vi "Init.vi"(8 "error in (no error)":errorcluster, 11 "LHL Actor in":refnum<class "LHL Actor.lvclass">) -> (0 "error out":errorcluster, 3 "LHL Actor out":refnum<class "LHL Actor.lvclass">)   [LabVIEW 2020, in "LHL Actor.lvlib" / "LHL Actor.lvclass"]
uses:
  LHL Actor.lvclass
  LHL Actor.lvclass/LHL Actor.ctl
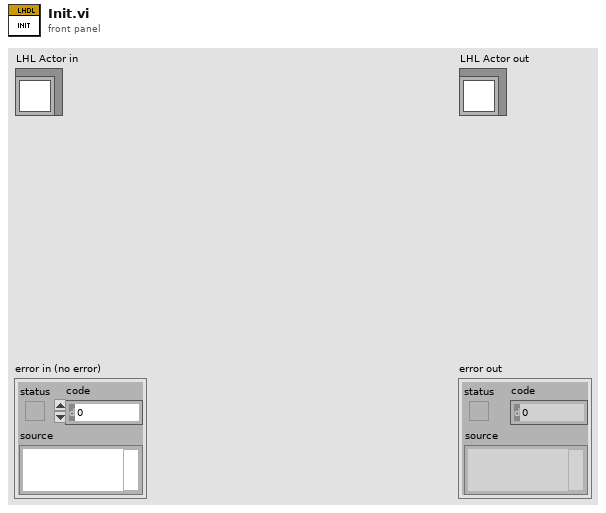
[diagram p1: front panel]
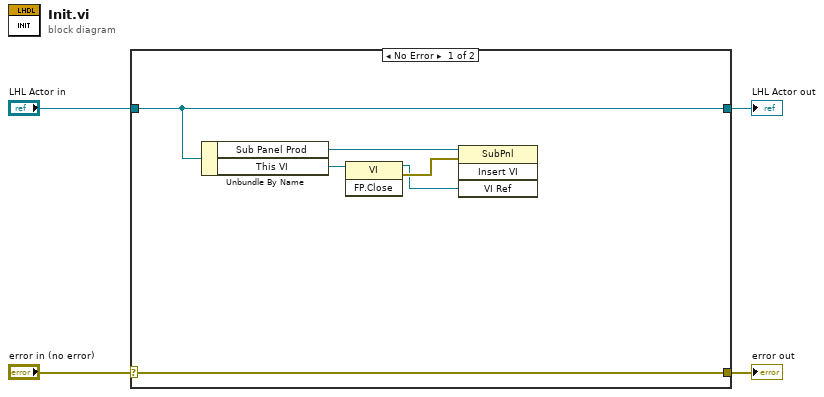
[diagram p0: block diagram]
diagram:
  n1 = case shown="No Error" "error in (no error)" {
    selector: "error in (no error)" -> [w10 w12]
    tunnel: [w10 w12] -> w3
    tunnel: [w5 w11] -> w1
    tunnel: "LHL Actor in" -> [w5 w11]
    frame No Error {
      n2 = Unbundle By Name(w5) -> ("Sub Panel Prod"=w6:refnum<vi>, "This VI"=w7:refnum<vi>)
      n3 = invoke class="VI" method="FP.Close"(reference=w7) -> (reference out=w8:refnum<vi>, error out=w9:errorcluster)  [unwired: 2 in, 1 out]
      n4 = invoke class="SubPnl" method="Insert VI"(reference=w6, error in=w9, "VI Ref"=w8) -> ()  [unwired: 1 in, 4 out]
    }
    frame Error {
    }
  }
  "error out" <- w3
  "LHL Actor out" <- w1
